vi "Log Rest and Release.vi"(8 "Error In":errorcluster, 9 "Timeout (s)":dbl=10.0 format="%#_13g", 11 "TDMS Log In":refnum<class "TDMS Logger.lvclass">) -> (0 "Error Out":errorcluster)   [LabVIEW 2014, in "TDMS Logger.lvlib" / "TDMS Logger.lvclass"]
doc: "This method will wait until all elements in the queue have been logged to files correctly and only then it will stop the asynchronous logger.\n\nUse this function to be sure that everything was logged before you stopped.\n\n<b>The default waiting time is 10s but you can wire any time at the imput. If there is a timeout an error 5789 will be thrown by this function. Handle this error in you application.</b>"
uses:
  TDMS Logger.lvclass
  _Typedefs/Log Message.ctl
  _Typedefs/Log Action.ctl
  _Typedefs/Data Type.ctl
  TDMS Logger.lvclass/TDMS Logger.ctl
  <vilib>/Utility/error.llb/Error Cluster From Error Code.vi
  <vilib>/ErrorRing/Error Ring.xnode
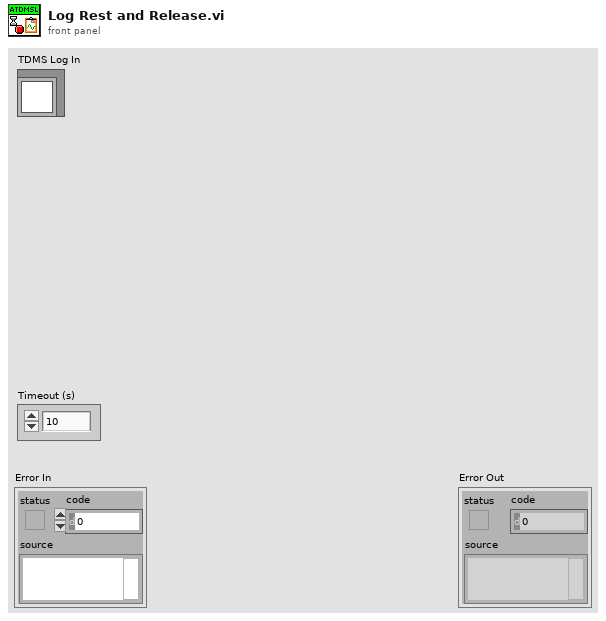
[diagram p1: front panel]
types:
  T1 = typedef "TDMS Logger.lvlib/TDMS Logger.lvclass/Log Action.ctl" = enum16{"Handle Old Files", "Status Update", "Stop", "Log Data", "Initialize"}
  T2 = typedef "TDMS Logger.lvlib/TDMS Logger.lvclass/Log Message.ctl" = cluster{"Log Action":T1, "Variant":variant, "Data Type":T3, "Group Name":string, "Channels Names":string[]}
  T3 = typedef "TDMS Logger.lvlib/TDMS Logger.lvclass/Data Type.ctl" = enum16{"I16", "I8", "String", "U16", "U8", "Waveform", "Double", "Single"}
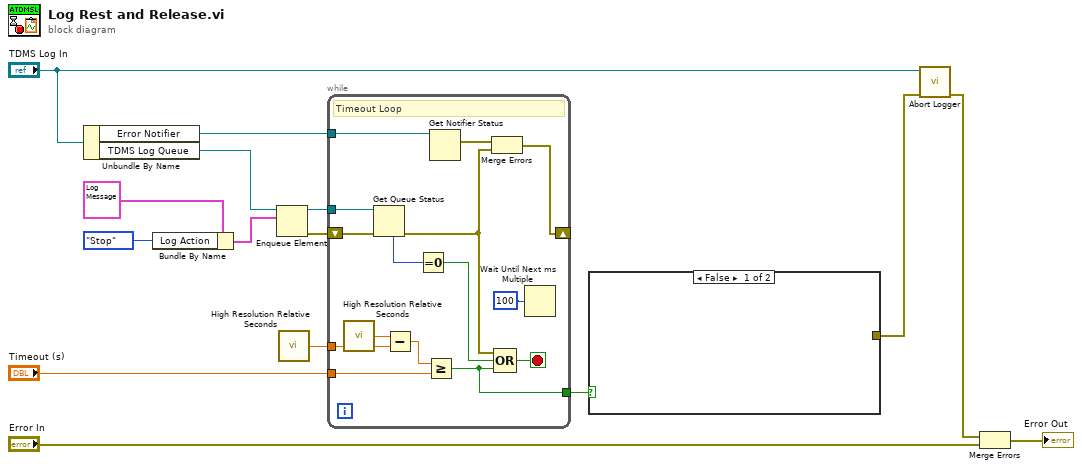
[diagram p0: block diagram]
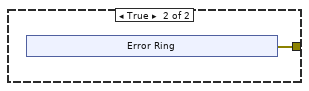
[diagram p2: hidden frame]
diagram:
  n1 = Unbundle By Name("TDMS Log In") -> ("Error Notifier"=w4:refnum<notifier>, "TDMS Log Queue"=w11:refnum<queue>)
  n2 = Bundle By Name(cluster=T2 {"Log Action"=enum."Handle Old Files", "Variant"=variant, "Data Type"=enum."String", "Group Name"="", "Channels Names"=[]} ("element"), "Log Action"=Log_Action."Stop") -> (w12:T2)
  n3 = Enqueue Element(queue=w11, element=w12) -> (queue out=w9:refnum<queue>, error out=w7:errorcluster)  [unwired: 2 in, 1 out]
  n4 = call <vilib>:"High Resolution Relative Seconds.vi"() -> ("relative seconds"=w8:dbl)
  n5 = while {
    tunnel: w9 -> [w30]
    tunnel: w8 -> [w27]
    tunnel: "Timeout (s)" -> [w24]
    tunnel: [w21] -> w6
    shift-right: [w16] -> _
    shift-left: w7 -> [w26]
    tunnel: w4 -> [w19]
    stop <- w22 stop-if-true
    # "Timeout Loop"
    n6 = call <vilib>:"High Resolution Relative Seconds.vi"() -> ("relative seconds"=w28:dbl)
    n7 = Get Queue Status(queue=w30, error in (no error)=w26) -> (error out=w17:errorcluster, # elements in queue=w29:i32)  [unwired: 1 in, 6 out]
    n8 = Subtract(x=w28, y=w27) -> (x-y=w25:dbl)
    n9 = Equal To 0?(x=w29) -> (x = 0?=w23:bool)
    n10 = Greater Or Equal?(x=w25, y=w24) -> (x >= y?=w21:bool)
    n11 = Get Notifier Status(notifier=w19) -> (current notification=w18:errorcluster)  [unwired: 1 in, 4 out]
    n12 = Merge Errors(w18, w17) -> (w16:errorcluster)
    n13 = Compound Arithmetic op=OR(w17, w23, w21) -> (w22:bool)
    n14 = Wait Until Next ms Multiple(millisecond multiple=u32 100) -> ()  [unwired: 1 out]
  }
  n15 = case shown="False" w6 {
    tunnel: [_ w31] -> w2
    frame False {
    }
    frame True {
      n16 = xnode "Error Ring"() -> ("error out"=w31:errorcluster)
    }
  }
  n17 = call "Abort Logger.vi"("Error In"=w2, "TDMS Log In"="TDMS Log In") -> ("Error Out"=w1:errorcluster)  [unwired: 9 in]
  n18 = Merge Errors(w1, "Error In") -> (→"Error Out":errorcluster)
